vi "K2000_init_fastseq.vi"(0 "GPIB address":string) -> ()   [LabVIEW 2013]
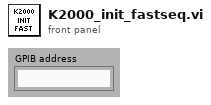
[diagram p1: front panel]
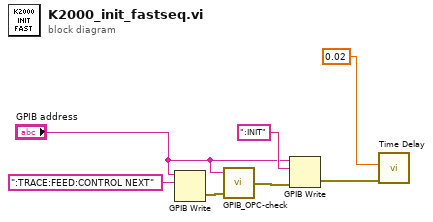
[diagram p0: block diagram]
diagram:
  n1 = GPIB Write(0:"GPIB address", 1:":TRACE:FEED:CONTROL NEXT" ("data")) -> (6:w7:errorcluster)  [unwired: 1 in, 3 out]
  n2 = call "GPIB_OPC-check.vi"("error out 2"=w7, "GPIB Address"="GPIB address") -> ("error out"=w6:errorcluster)  [unwired: 1 out]
  n3 = GPIB Write(0:"GPIB address", 1:":INIT" ("data string"), 3:w6) -> (6:w3:errorcluster)  [unwired: 3 out]
  n4 = call "Time Delay"("error in (no error)"=w3, "Delay Time (s)"=0.02) -> ()  [unwired: 10 out]
